vi "Init.vi"(5 "Client URI":refnum<class "URI.lvclass">, 6 "Session":refnum<class "Session.lvclass">, 7 "HTTPS?":bool, 8 "Values":refnum<class "Values.lvclass">, 9 "Server":refnum<class "Server.lvclass">, 10 "Trace Log":refnum<class "RequestTraceLog.lvclass">, 11 "TCP":refnum<k5>) -> (3 "Processing out":refnum<class "Processing.lvclass">)   [LabVIEW 2020, in "HTTP Server.lvlib" / "Processing.lvclass"]
uses:
  Processing.lvclass
  Processing.lvclass/Processing.ctl
  Server/Server.lvclass
  RequestTraceLog/RequestTraceLog.lvclass
  Values/Values.lvclass
  Session/Session.lvclass
  lv-uri/URI/URI/URI.lvclass
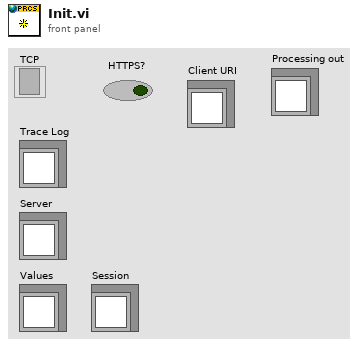
[diagram p1: front panel]
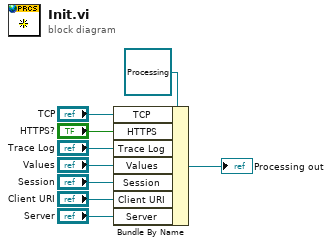
[diagram p0: block diagram]
diagram:
  n1 = Bundle By Name(cluster=refnum<class "Processing.lvclass"> refnum ("Processing in"), "TCP"="TCP", "HTTPS"="HTTPS?", "Trace Log"="Trace Log", "Values"="Values", "Session"="Session", "Client URI"="Client URI", "Server"="Server") -> (→"Processing out":refnum<class "Processing.lvclass">)
